vi "9871 EPICS - cRIO - Main Test1.vi"() -> ()   [LabVIEW 2021]
doc: "This is the top level VI for a cRIO target. This example will perform a read and a write from the same port on the 987x module. You can use this VI to verify that the port is working correctly. It uses two DMA channels for communication, one channel from the FPGA to the controller and one channel from the controller to the FPGA. For this reason a cRIO-900x contoller can not be used with this VI. You must use the other examples in this program as they only use DMA from the FPGA to the controller, which is supported by all cRIO controllers.\n\nPlease see the block diagram for more detailed comments."
uses:
  <vilib>/LabVIEW Targets/FPGA/cRIO/shared/nicrio_ModuleControls/nicrio_cRIO-9871_BaudRateEnum.ctl
  <vilib>/LabVIEW Targets/FPGA/cRIO/shared/nicrio_ModuleControls/nicrio_cRIO-9871_DataBitsEnum.ctl
  <vilib>/LabVIEW Targets/FPGA/cRIO/shared/nicrio_ModuleControls/nicrio_cRIO-9871_FlowControlEnum.ctl
  <vilib>/LabVIEW Targets/FPGA/cRIO/shared/nicrio_ModuleControls/nicrio_cRIO-9871_ParityEnum.ctl
  <vilib>/LabVIEW Targets/FPGA/cRIO/shared/nicrio_ModuleControls/nicrio_cRIO-9871_StopBitsEnum.ctl
  <vilib>/FPGAPlugInAG/cRIO-9047/niLvFpga_Open_cRIO-9047.vi
  <vilib>/FPGAPlugInAG/cRIO-9047/niLvFpga_Reset_cRIO-9047.vi
  <vilib>/FPGAPlugInAG/cRIO-9047/niLvFpga_Run_cRIO-9047.vi
  <vilib>/Utility/error.llb/Error Cluster From Error Code.vi
  <vilib>/rvi/errors/niLvFpgaAdjustHostInterfaceError.vi
  <vilib>/FPGAPlugInAG/cRIO-9047/niLvFpga_Close_cRIO-9047.vi
  <vilib>/rvi/interface/nirviOpenFPGA/nirviOpenFPGA.xnode
  FPGA Bitfiles/9871_EPICS_FPGA_Main_20230217.lvbitx
  <vilib>/rvi/interface/nirviMethod/nirviMethod.xnode
  <vilib>/rvi/interface/nirviReadWriteControl/nirviReadWriteControl.xnode
  <vilib>/rvi/interface/nirviCloseFPGA/nirviCloseFPGA.xnode
  <vilib>/rvi/errors/niLvFpgaMergeErrorWithErrorCode.vi
  NiFpgaLv.dll
  <vilib>/FPGAPlugInAG/cRIO-9047/niLvFpga_ReadFifo_cRIO-9047.vi
  <vilib>/FPGAPlugInAG/cRIO-9047/niLvFpga_WriteFifo_cRIO-9047.vi
panel:
  in  "Stop Bits":T1
  in  "Parity":T2
  in  "Flow Control":T3
  in  "Data Bits":T4=enum."8"
  in  "Baud Rate":T5=enum."9600 bps" caption="Baud"
  out "ReadPort":u16[](array[numeric])
  in  "Port# (1-4)":u8=1 min=1 max=4
  in  "Request Type":T6(ring)=enum."Echo Request"
  out "ReadData":u16[](array[numeric]) format="%016b"
  out "ReadError":errorcluster
  out "P3ReadError":errorcluster
  out "RX3FIFOTOCount":u32
  out "RX3ErrorCount":u32
  out "P4ReadError":errorcluster
  out "RX4FIFOTOCount":u32
  out "RX4ErrorCount":u32
  out "P2ReadError":errorcluster
  out "RX2FIFOTOCount":u32
  out "RX2ErrorCount":u32
  out "RX1FIFOTOCount":u32
  out "RX1ErrorCount":u32
  out "TXTOCount":u32
  out "TXErrorCount":u32
  out "P1ReadError":errorcluster
  out "WriteError":errorcluster
  in  "stop":bool
  in  "Write":bool
  out "WriteError":errorcluster
  out "WrBytesLeft":u32
  out "Elements Received":i32
  out "Receive String":string
  in  "Send String":string="ABCDEFGHIJKLMNOPQRSTUVWXYZ-abcdefghijklmnopqrstuvwxyz-0123456789"
  # "Transmit"
  # "Receive"
  # "Parameters"
  # "Write"
  # "Read"
  # "READ"
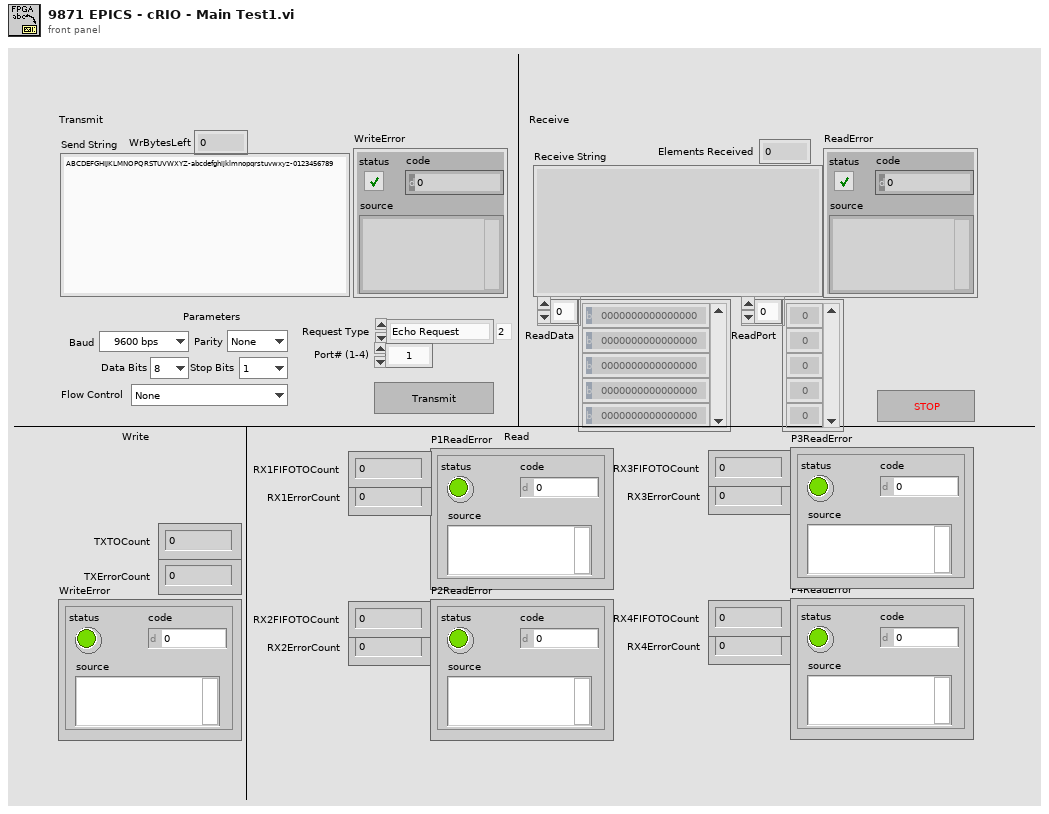
[diagram p1: front panel]
types:
  T1 = typedef "nicrio_cRIO-9871_StopBitsEnum.ctl" = enum8{"1", "1.5", "2"}
  T2 = typedef "nicrio_cRIO-9871_ParityEnum.ctl" = enum8{"None", "Odd", "Even", "Mark", "Space"}
  T3 = typedef "nicrio_cRIO-9871_FlowControlEnum.ctl" = enum8{"None", "Software (XON / XOFF)", "Hardware (RTS / CTS)"}
  T4 = typedef "nicrio_cRIO-9871_DataBitsEnum.ctl" = enum8{"5", "6", "7", "8"}
  T5 = typedef "nicrio_cRIO-9871_BaudRateEnum.ctl" = enum16{"75 bps", "110 bps", "134 bps", "150 bps", "300 bps", "600 bps", "1200 bps", "1800 bps", "2400 bps", "4800 bps", "7200 bps", "9600 bps", "14.4 kbps", "19.2 kbps", "28.8 kbps", "38.4 kbps", "57.6 kbps", "115.2 kbps", "230.4 kbps", "460.8 kbps", "921.6 kbps"}
  T6 = enum16{"TX Byte", "TX Clear", "Echo Request", "Parameter Change"}
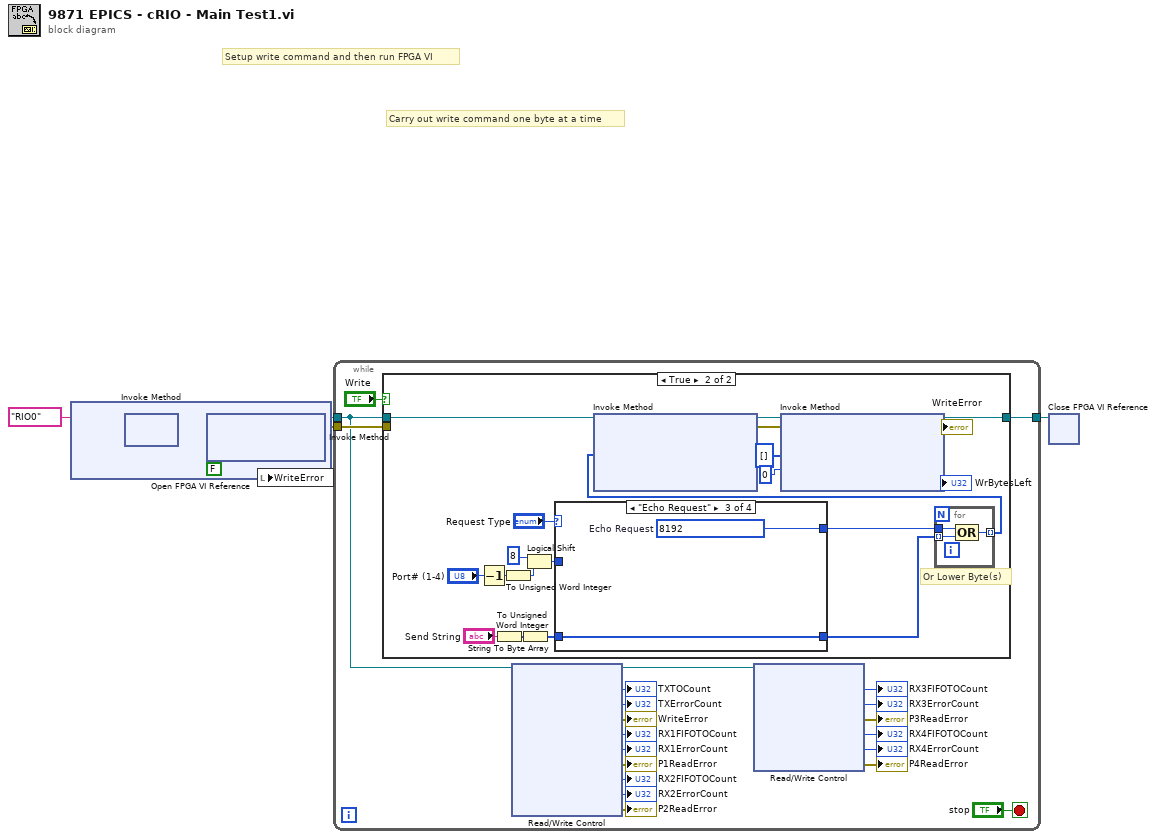
[diagram p0: block diagram]
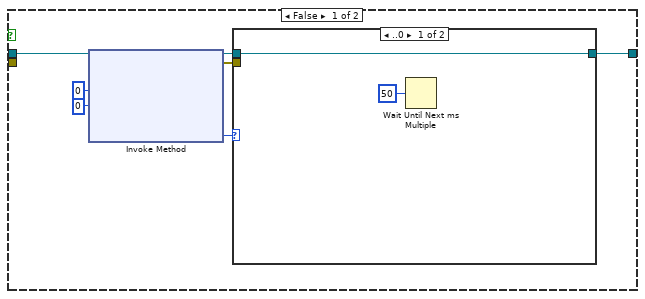
[diagram p2: hidden frame]
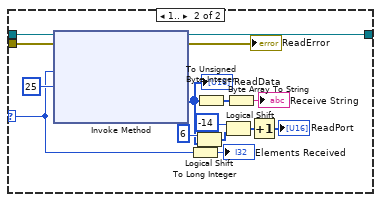
[diagram p3: hidden frame]
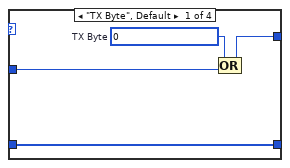
[diagram p4: hidden frame]
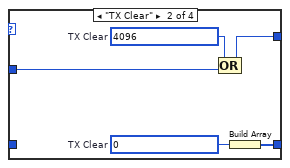
[diagram p5: hidden frame]
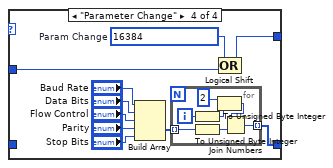
[diagram p6: hidden frame]
diagram:
  # "Carry out write command one byte at a time"
  # "Setup write command and then run FPGA VI"
  n1 = xnode "Open FPGA VI Reference"("resource name"=tag "RIO0") -> ("FPGA VI Reference Out"=w5:refnum<k20>, "error out"=w9:errorcluster)  [unwired: 1 in]
  n2 = xnode "Invoke Method"("FPGA VI Reference In"=w5, "error in"=w9) -> ("FPGA VI Reference Out"=w6:refnum<k20>, "error out"=w7:errorcluster)
  n3 = xnode "Invoke Method"("FPGA VI Reference In"=w6, "error in"=w7, "Wait Until Done (F)"=FALSE) -> ("FPGA VI Reference Out"=w3:refnum<k20>, "error out"=w4:errorcluster)
  n4 = local write "WriteError"(w4) -> ()
  n5 = while {
    tunnel: w4 -> [w30]
    tunnel: w3 -> [w11]
    tunnel: [w10] -> w2
    stop <- "stop" stop-if-true
    n6 = case shown="True" "Write" {
      tunnel: [w32 w70] -> w10
      tunnel: w11 -> [w33 w71]
      tunnel: w30 -> [_ _]
      frame False {
        n7 = xnode "Invoke Method"("FPGA VI Reference In"=w33, "Number of Elements"=u32 0, "Timeout (ms)"=0) -> ("FPGA VI Reference Out"=w36:refnum<k20>, "error out"=w37:errorcluster, "Elements Remaining"=w31:u32)  [unwired: 1 in, 1 out]
        n8 = case shown="..0" w31 {
          selector: w31 -> [_ w47]
          tunnel: w37 -> [_ w54]
          tunnel: w36 -> [w39 w53]
          tunnel: [w39 w48] -> w32
          frame ..0 {
            n9 = Wait Until Next ms Multiple(millisecond multiple=u32 50) -> ()  [unwired: 1 out]
          }
          frame 1.. {
            n10 = xnode "Invoke Method"("FPGA VI Reference In"=w53, "error in"=w54, "Number of Elements"=w47, "Timeout (ms)"=25) -> ("FPGA VI Reference Out"=w48:refnum<k20>, "error out"=→"ReadError":errorcluster, "Data"=w41:u16[])  [unwired: 1 out]
            "ReadData" <- w41
            n11 = To Long Integer(number=w47) -> (32bit integer=→"Elements Received":i32)
            n12 = Logical Shift(y=i16 6, x=w41) -> (x << y=w43:u16[])
            n13 = To Unsigned Byte Integer(number=w41) -> (unsigned 8bit integer=w52:u8[])
            n14 = Logical Shift(y=i16 -14, x=w43) -> (x << y=w42:u16[])
            n15 = Byte Array To String(unsigned byte array=w52) -> (string=→"Receive String":string)
            n16 = Increment(x=w42) -> (x+1=→"ReadPort":u16[])
          }
        }
      }
      frame True {
        # "Or Lower Byte(s)"
        n17 = Decrement(x="Port# (1-4)") -> (x-1=w60:u8)
        n18 = String To Byte Array(string="Send String") -> (unsigned byte array=w56:u8[])
        n19 = To Unsigned Word Integer(number=w60) -> (unsigned 16bit integer=w62:u16)
        n20 = To Unsigned Word Integer(number=w56) -> (unsigned 16bit integer=w55:u16[])
        n21 = Logical Shift(y=i16 8, x=w62) -> (x << y=w58:u16)
        n22 = case shown="\"Echo Request\"" "Request Type" {
          tunnel: [w77 w81 w85 w88] -> w63
          tunnel: w58 -> [w76 w83 _ w90]
          tunnel: [w75 w80 w84 w86] -> w57
          tunnel: w55 -> [w75 _ w84 _]
          frame "TX Byte", Default {
            w78 = u16 0  # TX Byte
            n23 = Compound Arithmetic op=OR(w78, w76) -> (w77:u16)
          }
          frame "TX Clear" {
            w79 = u16 0  # TX Clear
            w82 = u16 4096  # TX Clear
            n24 = Compound Arithmetic op=OR(w82, w83) -> (w81:u16)
            n25 = Build Array(w79) -> (w80:u16[])
          }
          frame "Echo Request" {
            w85 = u16 8192  # Echo Request
          }
          frame "Parameter Change" {
            w89 = u16 16384  # Param Change
            n26 = Build Array("Baud Rate", "Data Bits", "Flow Control", "Parity", "Stop Bits") -> (w87:u16[])
            n27 = for {
              tunnel: w87 -> [w102] mode=indexing
              tunnel: [w99] -> w86 mode=indexing
              i -> [w100]
              n28 = To Unsigned Byte Integer(number=w100) -> (unsigned 8bit integer=w96:u8)
              n29 = To Unsigned Byte Integer(number=w102) -> (unsigned 8bit integer=w101:u8)
              n30 = Logical Shift(y=i16 2, x=w96) -> (x << y=w97:u8)
              n31 = Join Numbers(hi=w97, lo=w101) -> ((hi.lo)=w99:u16)
            }
            n32 = Compound Arithmetic op=OR(w89, w90) -> (w88:u16)
          }
        }
        n33 = for {
          tunnel: w57 -> [w103] mode=indexing
          tunnel: [w105] -> w66 mode=indexing
          tunnel: w63 -> [w104]
          n34 = Compound Arithmetic op=OR(w104, w103) -> (w105:u16)
        }
        n35 = xnode "Invoke Method"("FPGA VI Reference In"=w71, "Data"=w66) -> ("FPGA VI Reference Out"=w72:refnum<k20>, "error out"=w69:errorcluster)  [unwired: 2 in, 1 out]
        n36 = xnode "Invoke Method"("FPGA VI Reference In"=w72, "error in"=w69, "Data"=u16[] [], "Timeout (ms)"=0) -> ("FPGA VI Reference Out"=w70:refnum<k20>, "error out"=→"WriteError":errorcluster, "Empty Elements Remaining"=→"WrBytesLeft":u32)
      }
    }
    n37 = xnode "Read/Write Control"("FPGA VI Reference In"=w11) -> ("FPGA VI Reference Out"=w27:refnum<k20>, "TXTOCount"=→"TXTOCount":u32, "TXErrorCount"=→"TXErrorCount":u32, "WriteError"=→"WriteError":errorcluster, "RX1FIFOTOCount"=→"RX1FIFOTOCount":u32, "RX1ErrorCount"=→"RX1ErrorCount":u32, "P1ReadError"=→"P1ReadError":errorcluster, "RX2FIFOTOCount"=→"RX2FIFOTOCount":u32, "RX2ErrorCount"=→"RX2ErrorCount":u32, "P2ReadError"=→"P2ReadError":errorcluster)  [unwired: 1 in, 1 out]
    n38 = xnode "Read/Write Control"("FPGA VI Reference In"=w27) -> ("RX3FIFOTOCount"=→"RX3FIFOTOCount":u32, "RX3ErrorCount"=→"RX3ErrorCount":u32, "P3ReadError"=→"P3ReadError":errorcluster, "RX4FIFOTOCount"=→"RX4FIFOTOCount":u32, "RX4ErrorCount"=→"RX4ErrorCount":u32, "P4ReadError"=→"P4ReadError":errorcluster)  [unwired: 1 in, 2 out]
  }
  n39 = xnode "Close FPGA VI Reference"("FPGA VI Reference In"=w2) -> ()  [unwired: 1 in, 1 out]
